vi "Volt Reader Trigger2.vi"() -> ()   [LabVIEW 2014]
uses:
  <vilib>/Utility/error.llb/DialogType.ctl
  <vilib>/_DAQmxBase/Internals/DAQmxBase Create Channel (AI-Voltage-Basic).vi
  <vilib>/_DAQmxBase/Internals/DAQmxBase Timing (Sample Clock).vi
  <vilib>/_DAQmxBase/Internals/DAQmxBase Read (Analog 2D DBL NChan NSamp).vi
panel:
  in  "Buffer":dbl
  in  "Threshold":dbl
  in  "units":i32(ring)=10348 items=["Volts"=10348, "From Custom Scale"=10065]
  in  "stop":bool
  out "Waveform Chart":waveform(dbl)(graph)
  in  "physical channels":tag
  in  "maximum value":dbl=5.0 format="%0.2f"
  in  "minimum value":dbl=-5.0 format="%0.2f"
  in  "rate":i32=1000 caption="Sample Rate"
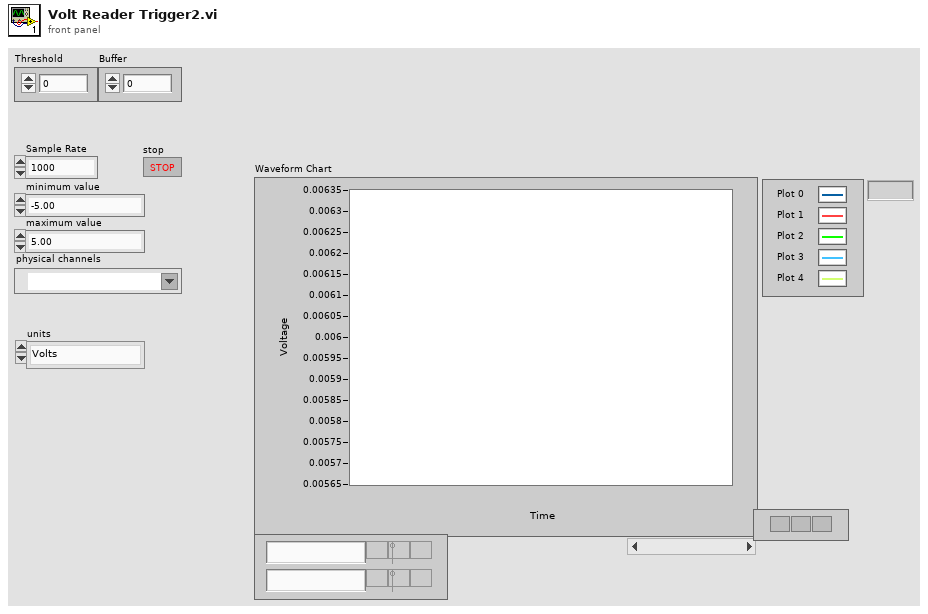
[diagram p1: front panel]
types:
  T1 = typedef "DialogType.ctl" = u16
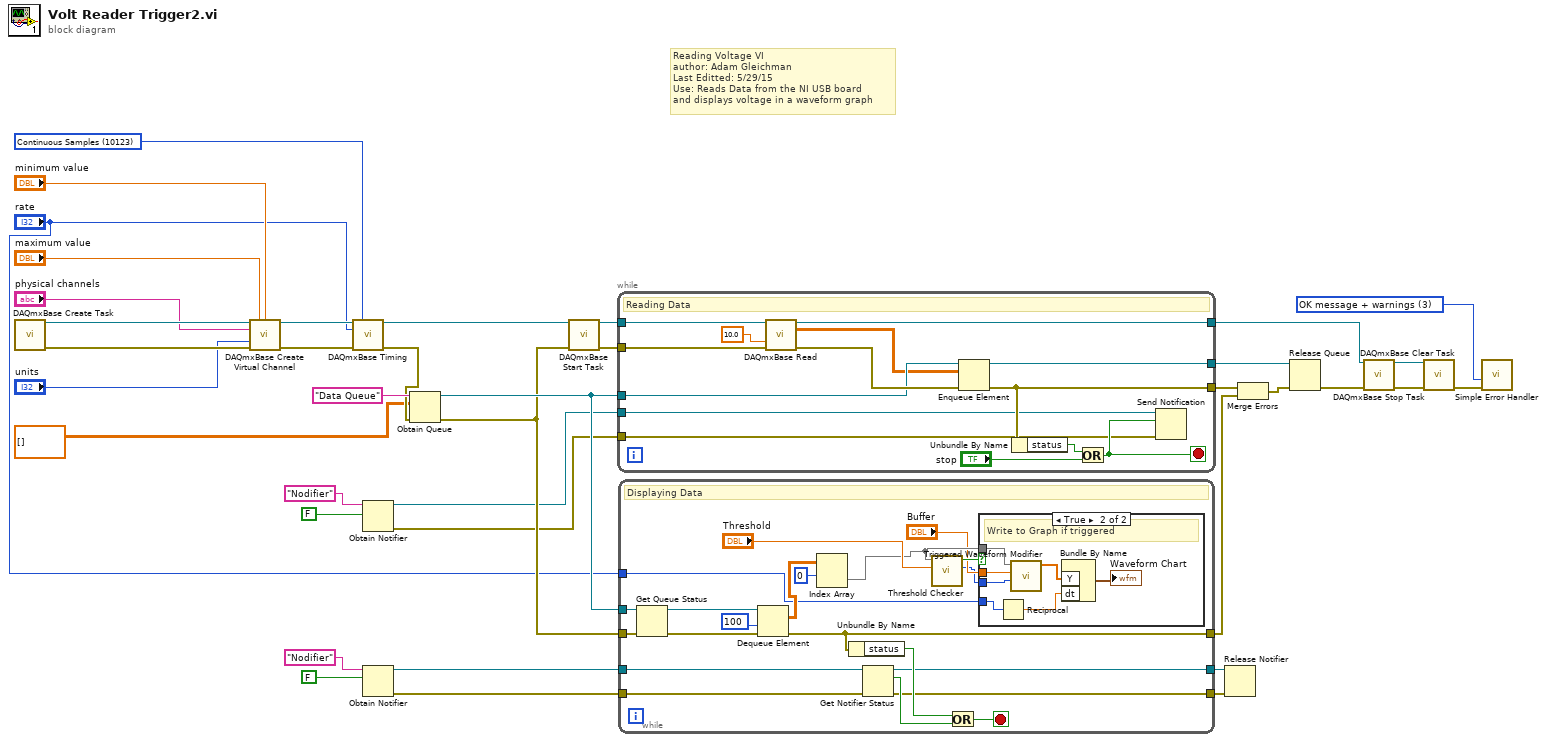
[diagram p0: block diagram]
diagram:
  w14 = 10123 items=["Finite Samples"=10178, "Continuous Samples"=10123, "Hardware Timed Single Point"=12522] ("sample mode")
  w16 = T1 3 items=["no dialog", "OK message", "continue or stop message", "OK message + warnings", "continue/stop + warnings"] ("type of dialog (OK msg:1)")
  # "Reading Voltage VI\nauthor: Adam Gleichman\nLast Editted: 5/29/15 \nUse: Reads Data from the NI USB board\nand displays voltage in a waveform graph"
  n1 = call <vilib>:"DAQmxBase Create Task.vi"() -> ("task out"=w37:refnum<k21>, "error out"=w36:errorcluster)  [unwired: 5 in, 9 out]
  n2 = call-poly <vilib>:"DAQmxBase Create Virtual Channel.vi"("task in"=w37, "maximum value"="maximum value", "minimum value"="minimum value", "physical channels"="physical channels", "units"="units", "error in"=w36) -> ("task out"=w34:refnum<k21>, "error out"=w35:errorcluster)  [unwired: 3 in, 5 out]
  n3 = call-poly <vilib>:"DAQmxBase Timing.vi"("task/channels in"=w34, "sample mode"=w14, "rate"="rate", "error in"=w35) -> ("task out"=w2:refnum<k21>, "error out"=w33:errorcluster)  [unwired: 3 in, 7 out]
  n4 = Obtain Notifier(name (unnamed)="Nodifier", notification data type=FALSE) -> (notifier out=w10:refnum<notifier>, error out=w9:errorcluster)  [unwired: 2 in, 1 out]
  n5 = Obtain Notifier(name (unnamed)="Nodifier", notification data type=FALSE) -> (notifier out=w7:refnum<notifier>, error out=w5:errorcluster)  [unwired: 2 in, 1 out]
  n6 = Obtain Queue(name (unnamed)="Data Queue", element data type=dbl[][] [] ("data"), error in (no error)=w33) -> (queue out=w23:refnum<queue>, error out=w22:errorcluster)  [unwired: 2 in, 1 out]
  n7 = call <vilib>:"DAQmxBase Start Task.vi"("task/channels in"=w2, "error in"=w22) -> ("task out"=w31:refnum<k21>, "error out"=w32:errorcluster)  [unwired: 12 out]
  n8 = while "Data Reading Loop" {
    tunnel: w32 -> [w51]
    tunnel: w31 -> [w52]
    tunnel: w23 -> [w49]
    tunnel: [w46] -> w26
    tunnel: [w44] -> w25
    tunnel: [w42] -> w13
    tunnel: w10 -> [w40]
    tunnel: w9 -> [w39]
    stop <- w41 stop-if-true
    # "Reading Data"
    n9 = call-poly <vilib>:"DAQmxBase Read.vi"("task/channels in"=w52, "timeout"=10.0, "error in"=w51) -> ("task out"=w42:refnum<k21>, "data"=w47:dbl[][], "error out"=w50:errorcluster)  [unwired: 10 in]
    n10 = Enqueue Element(queue=w49, element=w47, error in (no error)=w50) -> (queue out=w46:refnum<queue>, error out=w44:errorcluster)  [unwired: 1 in, 1 out]
    n11 = Unbundle By Name(w44) -> ("status"=w43:bool)
    n12 = Or(x=w43, y="stop") -> (x .or. y?=w41:bool)
    n13 = Send Notification(notification=w41, notifier=w40, error in (no error)=w39) -> ()  [unwired: 2 out]
  }
  n14 = while {
    tunnel: w23 -> [w73]
    tunnel: w22 -> [w62]
    tunnel: [w71] -> w21
    tunnel: w7 -> [w68]
    tunnel: w5 -> [w67]
    tunnel: [w65] -> w3
    tunnel: [w64] -> w4
    tunnel: "rate" -> [w53]
    stop <- w69 stop-if-true
    # "Displaying Data"
    n15 = Get Queue Status(queue=w73, error in (no error)=w62) -> (queue out=w63:refnum<queue>, error out=w61:errorcluster)  [unwired: 1 in, 6 out]
    n16 = Dequeue Element(queue=w63, timeout in ms (-1)=100, error in (no error)=w61) -> (element=w57:dbl[][], error out=w71:errorcluster)  [unwired: 2 out]
    n17 = Index Array(array=w57, index (row)=0 ("index")) -> (element=w56:dbl[])  [unwired: 1 in]
    n18 = Unbundle By Name(w71) -> ("status"=w70:bool)
    n19 = Get Notifier Status(notifier=w68, error in (no error)=w67) -> (notifier out=w65:refnum<notifier>, current notification=w66:bool, error out=w64:errorcluster)  [unwired: 2 out]
    n20 = call "Threshold Checker.vi"("Threshold"="Threshold", "Data"=w56) -> ("Index of Value = to or exceeding threshold"=w54:i32, "Did we pass the threshold?"=w58:bool)  [unwired: 7 in, 1 out]
    n21 = Or(x=w70, y=w66) -> (x .or. y?=w69:bool)
    n22 = case shown="True" w58 {
      tunnel: w56 -> [_ w80]
      tunnel: "Buffer" -> [_ w79]
      tunnel: w54 -> [_ w78]
      tunnel: w53 -> [_ w76]
      frame False {
        # "Write nothing on the graph"
      }
      frame True {
        # "Write to Graph if triggered"
        n23 = Reciprocal(x=w76) -> (1/x=w75:dbl)
        n24 = call "Triggered Waveform Modifier.vi"("Index"=w78, "Buffer"=w79, "Input Y Values"=w80) -> ("appended array"=w77:dbl[])  [unwired: 8 in]
        n25 = Bundle By Name("Y"=w77, "dt"=w75) -> (→"Waveform Chart":waveform(dbl))  [unwired: 1 in]
      }
    }
  }
  n26 = Release Notifier(notifier=w3, error in (no error)=w4) -> ()  [unwired: 1 in, 3 out]
  n27 = Merge Errors(w25, w21) -> (w24:errorcluster)
  n28 = Release Queue(queue=w26, error in (no error)=w24) -> (error out=w20:errorcluster)  [unwired: 1 in, 2 out]
  n29 = call <vilib>:"DAQmxBase Stop Task.vi"("task/channels in"=w13, "error in"=w20) -> ("task out"=w19:refnum<k21>, "error out"=w18:errorcluster)  [unwired: 12 in]
  n30 = call <vilib>:"DAQmxBase Clear Task.vi"("task in"=w19, "error in"=w18) -> ("error out"=w17:errorcluster)  [unwired: 13 in]
  n31 = call <vilib>:"Simple Error Handler.vi"("type of dialog (OK msg:1)"=w16, "error in (no error)"=w17) -> ()  [unwired: 3 in, 5 out]
